vi "setData.vi"(8 "error in (no error)":errorcluster, 10 "Data":string, 11 "Data in":refnum<class "Data.lvclass">) -> (0 "error out":errorcluster, 3 "Data out":refnum<class "Data.lvclass">)   [LabVIEW 2017, in "Filled Text Fields Actor.lvlib" / "Data.lvclass"]
uses:
  Data.lvclass
  Data.lvclass/Data.ctl
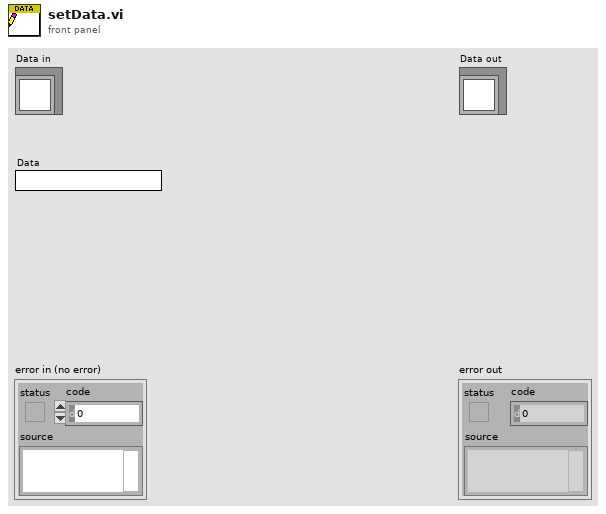
[diagram p1: front panel]
types:
  T1 = typedef "Filled Text Fields Actor.lvlib/Data.lvclass/Data.PrivateData.ctl" = cluster{"Data":string}
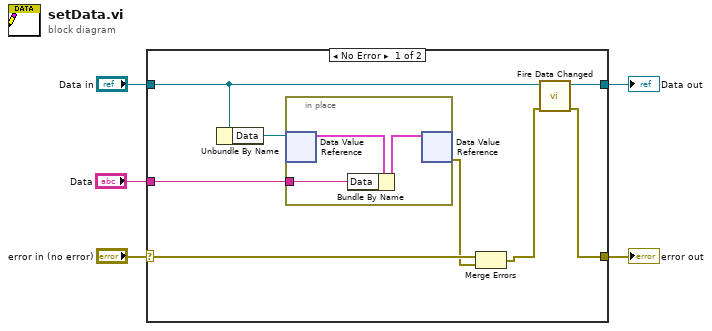
[diagram p0: block diagram]
diagram:
  n1 = case shown="No Error" "error in (no error)" {
    selector: "error in (no error)" -> [w13 w17]
    tunnel: [w6 w17] -> w4
    tunnel: [w8 w18] -> w2
    tunnel: "Data in" -> [w11 w18]
    tunnel: "Data" -> [w10 _]
    frame No Error {
      n2 = Unbundle By Name(w11) -> ("Data"=w12:refnum<data-value>)
      n3 = in-place {
        in-place-border: w10 -> [w14]
        n4 = in-place-dvr #1(w12) -> (w16:T1)  [unwired: 1 out]
        n5 = Bundle By Name(cluster=w16, "Data"=w14) -> (w15:T1)
        n6 = in-place-dvr #1(w15) -> (w9:errorcluster)  [unwired: 1 out]
      }
      n7 = Merge Errors(w13, w9) -> (w7:errorcluster)
      n8 = call "Fire Data Changed.vi"("error in (no error)"=w7, "Data in"=w11) -> ("error out"=w6:errorcluster, "Data out"=w8:refnum<class "Data.lvclass">)  [unwired: 8 in]
    }
    frame Error {
    }
  }
  "error out" <- w4
  "Data out" <- w2
